vi "Write SA Pin.vi"(8 "error in (no error)":errorcluster, 10 "SA Pin":string, 11 "NR_SEM in":refnum<class "NR_SEM.lvclass">) -> (0 "error out":errorcluster, 3 "NR_SEM out":refnum<class "NR_SEM.lvclass">)   [LabVIEW 2018, in "SeqAuto Evaluations.lvlib" / "NR_SEM.lvclass"]
uses:
  NR_SEM.lvclass
  NR_SEM.lvclass/NR_SEM.ctl
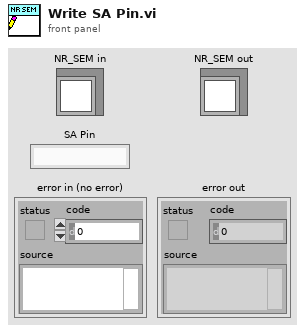
[diagram p1: front panel]
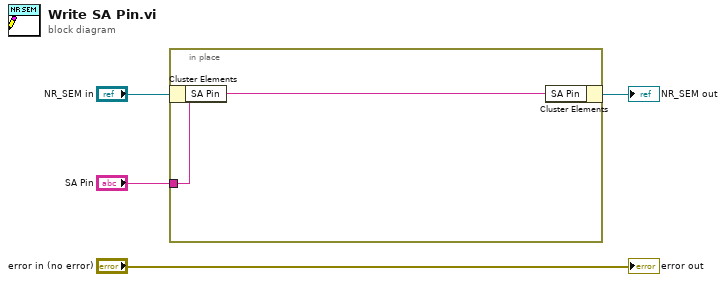
[diagram p0: block diagram]
diagram:
  n1 = in-place {
    in-place-border: "SA Pin" -> [w5]
    n2 = in-place-cluster #1("NR_SEM in") -> ()  [unwired: 1 out]
    n3 = in-place-cluster #1("SA Pin"=w5) -> (→"NR_SEM out":refnum<class "NR_SEM.lvclass">)
  }
  "error out" <- "error in (no error)"
